vi "ifr2025 Define.vi"(7 "Stop (0)":i16 format="%.0g", 8 "error in (no error)":errorcluster {"code" format="%.0x"}, 9 "Start (0)":i16 format="%.0g", 10 "Set (SEQ1)":i16(ring)=1 items=["SEQ1"=1, "SEQ2"=2, "SEQ3"=3, "SEQ4"=4, "SEQ5"=5, "SEQ6"=6, "SEQ7"=7, "SEQ8"=8, "SEQ9"=9], 11 "instrument handle":refnum<visa-resource-name>) -> (0 "error out":errorcluster {"code" format="%.0x"}, 3 "instrument handle out":refnum<visa-resource-name>)   [LabVIEW 2009]
doc: "This command allows up to 9 sequences, each consisting of a range of memory locations to be defined."
uses:
  Ifr2025_32.dll
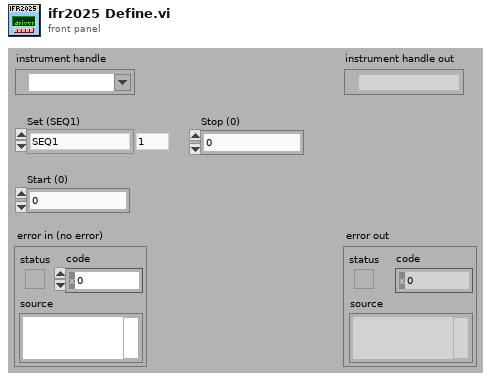
[diagram p1: front panel]
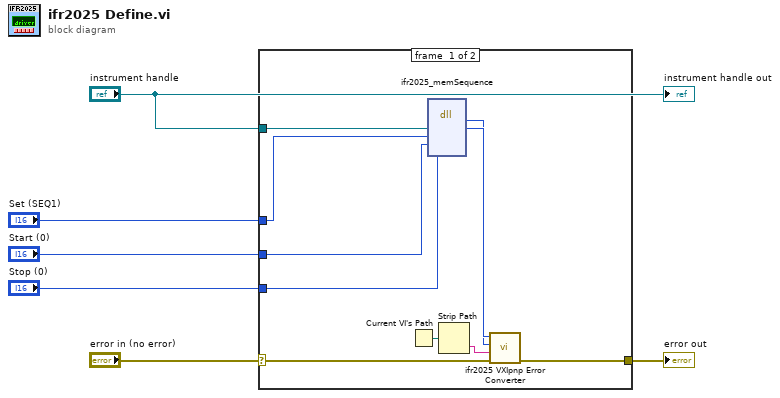
[diagram p0: block diagram]
diagram:
  n1 = case shown="No Error" "error in (no error)" {
    selector: "error in (no error)" -> [w11 w17]
    tunnel: [w10 w17] -> w6
    tunnel: "instrument handle" -> [w15 _]
    tunnel: "Set (SEQ1)" -> [w9 _]
    tunnel: "Start (0)" -> [w8 _]
    tunnel: "Stop (0)" -> [w7 _]
    frame #0 {
      n2 = Current VI's Path() -> (path=w16:path)
      n3 = dll-call lib="P:/inst/Marconi 2024 Signal Generator/source/labview/ifr2025/ifr2025/ifr2025_*.*" fn="ifr2025_memSequence"("vi"=w15, "Set"=w9, "Start"=w8, "Stop"=w7) -> (w13:i32, "vi"=w14:u32)  [unwired: 6 in, 2 out]
      n4 = Strip Path(path=w16) -> (name=w12:string)  [unwired: 1 out]
      n5 = call "ifr2025 VXIpnp Error Converter.vi"("error in (no error)"=w11, "name of VI (\"\")"=w12, "CVI error code (0)"=w13, "instrument handle"=w14) -> ("error out"=w10:errorcluster)  [unwired: 7 out]
    }
    frame #1 {
    }
  }
  "error out" <- w6
  "instrument handle out" <- "instrument handle"
